vi "IsEmptyListCtrl.vi"(11 "testcaseList":refnum<vi>) -> (3 "is empty?":bool)   [LabVIEW 2018, in "Library-Ctrl.lvlib"]
uses:
  Library-Ctrl.lvlib
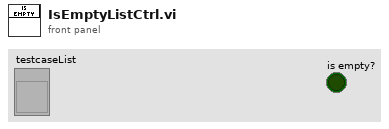
[diagram p1: front panel]
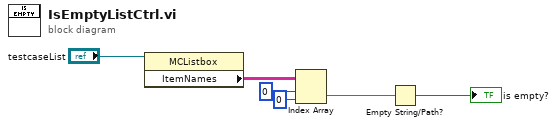
[diagram p0: block diagram]
diagram:
  n1 = property class="MCListbox"(reference="testcaseList") -> ("ItemNames"=w4:string[][])  [unwired: 1 in, 2 out]
  n2 = Index Array(array=w4, index (row)=0 ("인덱스 (행)"), index (col)=0 ("비활성화된 인덱스 (열)")) -> (element=w1:string)
  n3 = Empty String/Path?(string/path=w1) -> (empty?=→"is empty?":bool)
